vi "wfm_feature set_mouse_state.vi"(7 "mouse event":T1, 8 "error in (no error)":errorcluster, 11 "WindowGraph in":refnum<class "wfm_feature.lvclass">) -> (0 "error out":errorcluster, 3 "WindowGraph out":refnum<class "wfm_feature.lvclass">)   [LabVIEW 2018, in "wfm_feature.lvclass"]
uses:
  wfm_feature.lvclass
  subVI/mouse_state.ctl
  wfm_feature.lvclass/wfm_feature.ctl
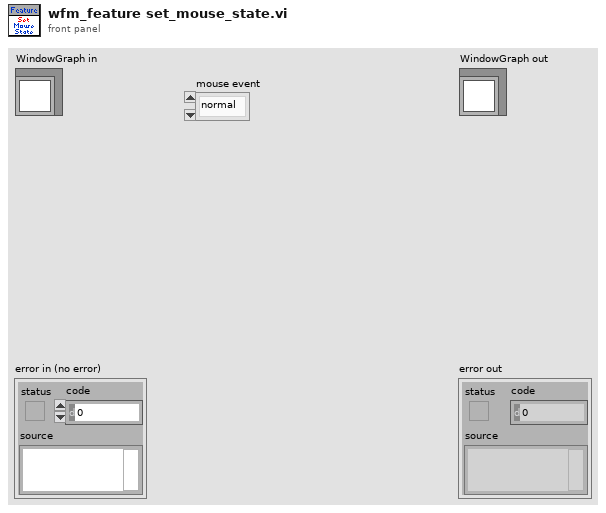
[diagram p1: front panel]
types:
  T1 = typedef "mouse_state.ctl" = enum16{"normal", "mouse down", "calc"}
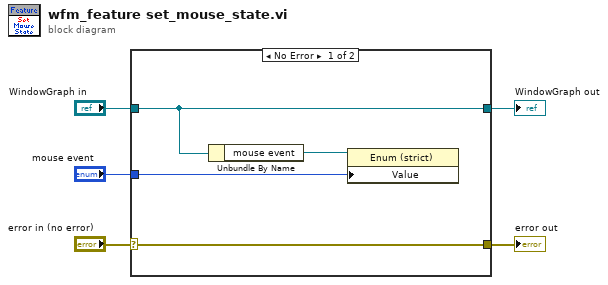
[diagram p0: block diagram]
diagram:
  n1 = case shown="No Error" "error in (no error)" {
    selector: "error in (no error)" -> [w9 w11]
    tunnel: [w9 w11] -> w4
    tunnel: [w8 w10] -> w2
    tunnel: "WindowGraph in" -> [w8 w10]
    tunnel: "mouse event" -> [w6 _]
    frame No Error {
      n2 = Unbundle By Name(w8) -> ("mouse event"=w7:refnum<vi>)
      n3 = property class="Enum (strict)"(reference=w7, "Value"=w6) -> ()  [unwired: 1 in, 2 out]
    }
    frame Error {
    }
  }
  "error out" <- w4
  "WindowGraph out" <- w2
